vi "Keithley6430subVI_V2.vi"(1 "K-6430 info in":T1) -> (7 "K6430 Measurement":dbl, 8 "K6430 info out":T1, 9 "K6430 measuremnet string":string)   [LabVIEW 2014]
uses:
  Drivers and Software/keithley_6430/Keithley 6430/Public/Data/Read (Single Point).vi
  Drivers and Software/keithley_6430/Keithley 6430/Keithley 6430.lvlib
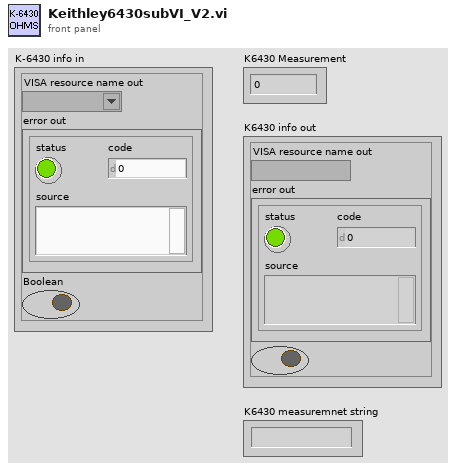
[diagram p1: front panel]
types:
  T1 = cluster{"VISA resource name out":refnum<visa-resource-name>, "error out":errorcluster, "Boolean":bool}
  T2 = cluster{"VISA resource name out":refnum<visa-resource-name>, "error out":errorcluster, bool}
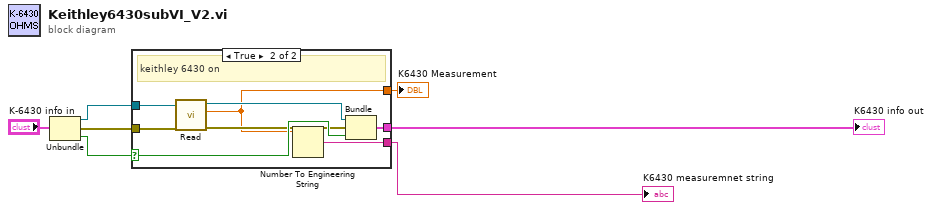
[diagram p0: block diagram]
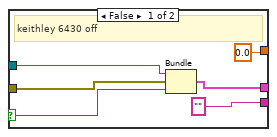
[diagram p2: hidden frame]
diagram:
  n1 = Unbundle("K-6430 info in") -> ("VISA resource name out"=w2:refnum<visa-resource-name>, "error out"=w3:errorcluster, "Boolean"=w4:bool)
  n2 = case "Keithley 6430" shown="True" w4 {
    selector: w4 -> [w11 w18]
    tunnel: w2 -> [w12 w20]
    tunnel: w3 -> [w9 w19]
    tunnel: ["" w21] -> w5
    tunnel: [w10 w15] -> w6
    tunnel: [0.0 ("Measurement") w14] -> w7
    frame False {
      # "keithley 6430 off"
      n3 = Bundle("VISA resource name out"=w12, "error out"=w9, w11) -> (w10:T2)  [unwired: 1 in]
    }
    frame True {
      # "keithley 6430 on"
      n4 = call-poly "Read.vi"("error in (no error)"=w19, "VISA resource name"=w20) -> ("error out"=w17:errorcluster, "Measurement"=w14:dbl, "VISA resource name out"=w16:refnum<visa-resource-name>)  [unwired: 1 in, 6 out]
      n5 = Number To Engineering String(4:w14) -> (0:w21:string)  [unwired: 3 in]
      n6 = Bundle("VISA resource name out"=w16, "error out"=w17, w18) -> (w15:T2)  [unwired: 1 in]
    }
  }
  "K6430 Measurement" <- w7
  "K6430 info out" <- w6
  "K6430 measuremnet string" <- w5
